vi "New.vi"(7 "CreateMethod(Create or look up existing)":T1(ring), 8 "error in (no error)":errorcluster, 10 "Object name":string, 11 "Websocket In":refnum<class "Websocket.lvclass">) -> (0 "error out":errorcluster, 1 "NewObjectCreated":bool, 2 "DVRRefOut":refnum<data-value>, 3 "Websocket Out":refnum<class "Websocket.lvclass">, 5 "ObjectQueueName":string)   [LabVIEW 2017, in "Front Panel Publisher.lvlib" / "Websocket.lvclass"]
uses:
  Websocket.lvclass
  Protected/Object Attributes.ctl
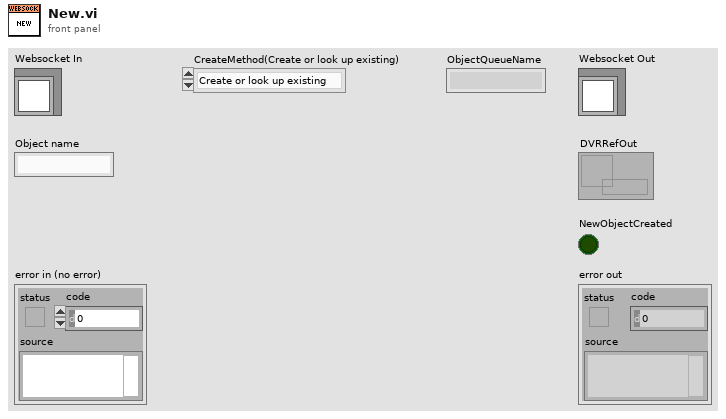
[diagram p1: front panel]
types:
  T1 = enum16{"Create or look up existing", "Look up existing"}
  T2 = typedef "Front Panel Publisher.lvlib/Websocket.lvclass/Object Attributes.ctl" = cluster{"Port":u16, "TCP Refs":refnum<k5>[], "Connection IDs":u64[]}
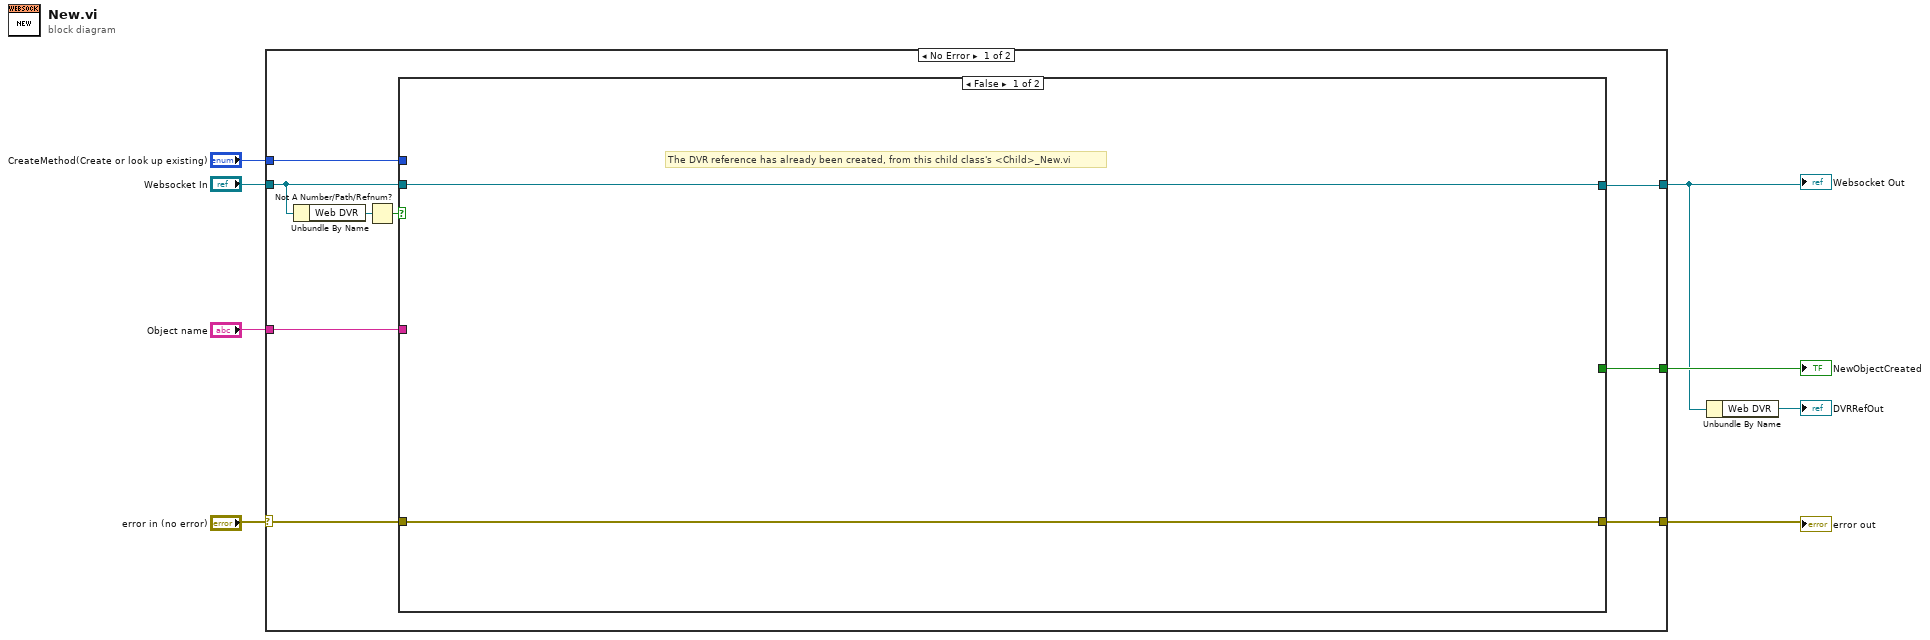
[diagram p0: block diagram]
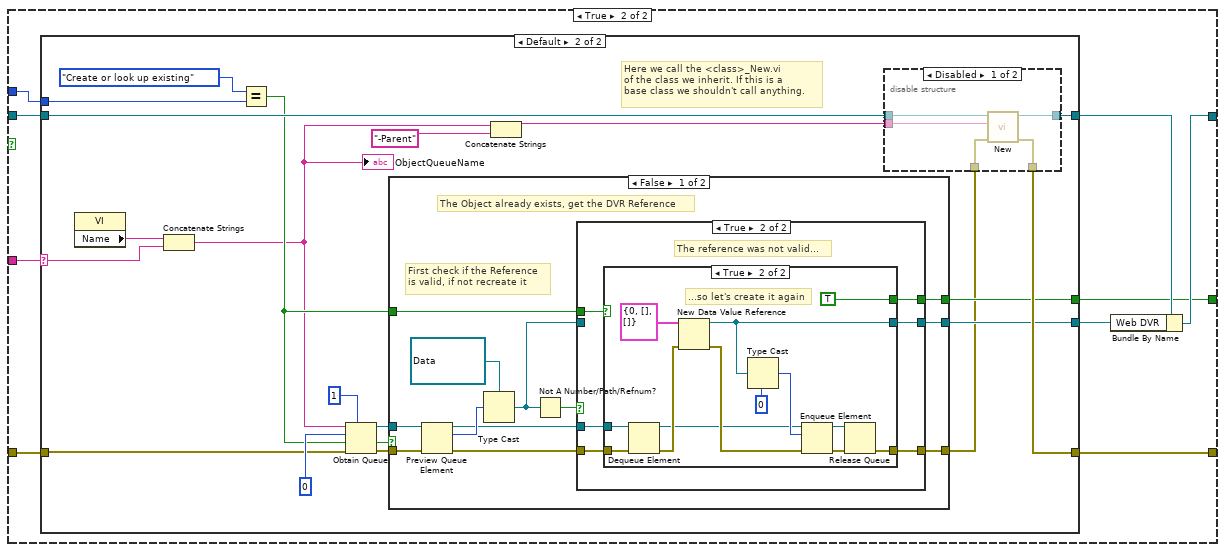
[diagram p2: hidden frame]
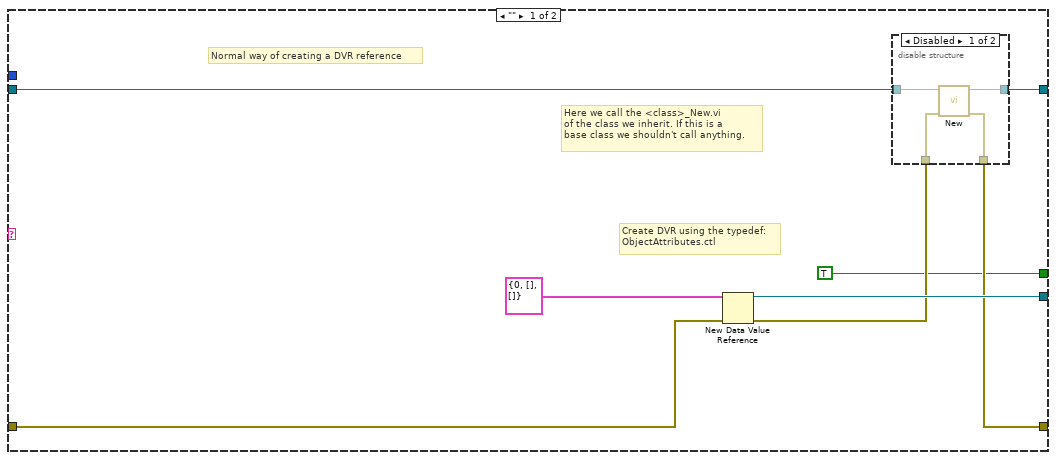
[diagram p3: hidden frame]
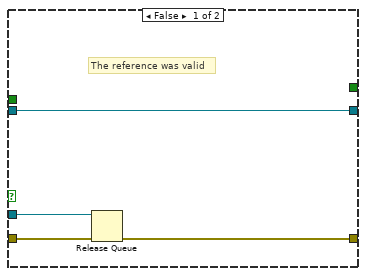
[diagram p5: hidden frame]
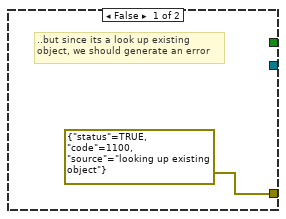
[diagram p6: hidden frame]
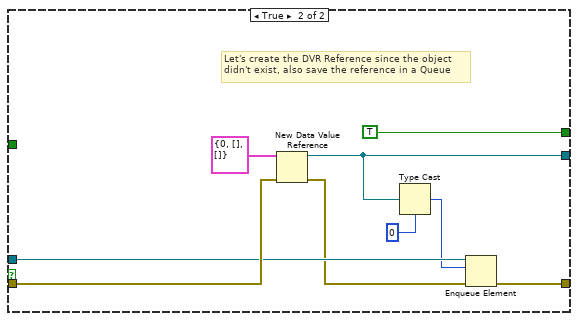
[diagram p7: hidden frame]
diagram:
  n1 = case shown="No Error" "error in (no error)" {
    selector: "error in (no error)" -> [w17 w116]
    tunnel: [w14 w116] -> w4
    tunnel: "CreateMethod(Create or look up existing)" -> [w15 _]
    tunnel: "Object name" -> [w16 _]
    tunnel: "Websocket In" -> [w13 w115]
    tunnel: [w12 w115] -> w2
    tunnel: [w11 _] -> w3
    frame No Error {
      n2 = Unbundle By Name(w13) -> ("Web DVR"=w10:refnum<data-value>)
      n3 = Not A Number/Path/Refnum?(number/path/refnum=w10) -> (NaN/Path/Refnum?=w9:bool)
      n4 = case shown="False" w9 {
        tunnel: w17 -> [w19 w28]
        tunnel: w16 -> [_ w27]
        tunnel: w15 -> [_ w26]
        tunnel: [w19 w25] -> w14
        tunnel: w13 -> [w18 w23]
        tunnel: [w18 w24] -> w12
        tunnel: [_ w21] -> w11
        frame False {
          # "The DVR reference has already been created, from this child class's <Child>_New.vi"
        }
        frame True {
          n5 = case shown="Default" w27 {
            selector: w27 -> [_ w54]
            tunnel: w28 -> [w36 w52]
            tunnel: [w31 w53] -> w25
            tunnel: w26 -> [_ w61]
            tunnel: [w35 w47] -> w20
            tunnel: w23 -> [w34 w60]
            tunnel: [w33 w59] -> w22
            tunnel: [TRUE w46] -> w21
            frame "" {
              # "Create DVR using the typedef:\nObjectAttributes.ctl"
              # "Here we call the <class>_New.vi\nof the class we inherit. If this is a\nbase class we shouldn't call anything."
              # "Normal way of creating a DVR reference"
              n6 = New Data Value Reference(data value=T2 {"Port"=0, "TCP Refs"=[], "Connection IDs"=[]} ("Data 2"), error in=w36) -> (data value reference=w35:refnum<data-value>, error out=w32:errorcluster)
              n7 = disable-structure shown="Disabled" {
                disable-tunnel: w34 -> [w40 w42]
                disable-tunnel: [w39 w42] -> w33
                disable-tunnel: w32 -> [w38 w41]
                disable-tunnel: [w37 w41] -> w31
                frame Disabled {
                  n8 = call "New.vi"("error in (no error)"=w38, "Websocket In"=w40) -> ("error out"=w37:errorcluster, "Websocket Out"=w39:refnum<class "Websocket.lvclass">)  [unwired: 5 in, 3 out]
                }
                frame Enabled {
                }
              }
            }
            frame Default {
              # "Here we call the <class>_New.vi\nof the class we inherit. If this is a\nbase class we shouldn't call anything."
              n9 = property class="VI"() -> ("Name"=w55:string)  [unwired: 2 in, 2 out]
              n10 = Concatenate Strings(w55, w54) -> (w43:string)
              "ObjectQueueName" <- w43
              n11 = Equal?(x=T1."Create or look up existing", y=w61) -> (x = y?=w48:bool)
              n12 = Obtain Queue(max queue size (-1, unlimited)=1, name (unnamed)=w43, element data type=u32 0 ("DataRef"), create if not found? (T)=w48, error in (no error)=w52) -> (queue out=w49:refnum<queue>, created new?=w50:bool, error out=w51:errorcluster)
              n13 = case shown="False" w50 {
                tunnel: w51 -> [w73 w107]
                tunnel: w49 -> [w74 w106]
                tunnel: [w69 w103] -> w45
                tunnel: [w67 w102] -> w47
                tunnel: [w65 TRUE] -> w46
                tunnel: w48 -> [w64 _]
                frame False {
                  # "First check if the Reference\nis valid, if not recreate it"
                  # "The Object already exists, get the DVR Reference"
                  n14 = Preview Queue Element(queue=w74, error in (no error)=w73) -> (queue out=w66:refnum<queue>, element=w72:u32, error out=w71:errorcluster)  [unwired: 1 in, 1 out]
                  n15 = Type Cast(type=refnum<data-value> refnum ("DVRRef(Hidden)"), x=w72) -> (*(type *) &x=w68:refnum<data-value>)
                  n16 = Not A Number/Path/Refnum?(number/path/refnum=w68) -> (NaN/Path/Refnum?=w70:bool)
                  n17 = case shown="True" w70 {
                    tunnel: w71 -> [w75 w83]
                    tunnel: [w76 w81] -> w69
                    tunnel: w68 -> [w78 _]
                    tunnel: [w78 w82] -> w67
                    tunnel: w66 -> [w77 w84]
                    tunnel: [_ w80] -> w65
                    tunnel: w64 -> [_ w79]
                    frame False {
                      # "The reference was valid"
                      n18 = Release Queue(queue=w77, error in (no error)=w75) -> (error out=w76:errorcluster)  [unwired: 1 in, 2 out]
                    }
                    frame True {
                      # "The reference was not valid..."
                      n19 = case shown="True" w79 {
                        tunnel: w84 -> [_ w98]
                        tunnel: w83 -> [_ w97]
                        tunnel: [_ w91] -> w82
                        tunnel: [errorcluster {"status"=TRUE, "code"=1100, "source"="looking up existing object"} ("error out") w87] -> w81
                        tunnel: [_ TRUE] -> w80
                        frame False {
                          # "..but since its a look up existing\nobject, we should generate an error"
                        }
                        frame True {
                          # "...so let's create it again"
                          n20 = Dequeue Element(queue=w98, error in (no error)=w97) -> (queue out=w92:refnum<queue>, error out=w94:errorcluster)  [unwired: 1 in, 2 out]
                          n21 = New Data Value Reference(data value=T2 {"Port"=0, "TCP Refs"=[], "Connection IDs"=[]} ("Data"), error in=w94) -> (data value reference=w91:refnum<data-value>, error out=w93:errorcluster)
                          n22 = Type Cast(type=u32 0 ("ObjectQueue"), x=w91) -> (*(type *) &x=w95:u32)
                          n23 = Enqueue Element(queue=w92, element=w95, error in (no error)=w93) -> (queue out=w88:refnum<queue>, error out=w89:errorcluster)  [unwired: 1 in, 1 out]
                          n24 = Release Queue(queue=w88, error in (no error)=w89) -> (error out=w87:errorcluster)  [unwired: 1 in, 2 out]
                        }
                      }
                    }
                  }
                }
                frame True {
                  # "Let's create the DVR Reference since the object\ndidn't exist, also save the reference in a Queue"
                  n25 = New Data Value Reference(data value=T2 {"Port"=0, "TCP Refs"=[], "Connection IDs"=[]} ("Data"), error in=w107) -> (data value reference=w102:refnum<data-value>, error out=w104:errorcluster)
                  n26 = Type Cast(type=u32 0 ("ObjectQueue"), x=w102) -> (*(type *) &x=w101:u32)
                  n27 = Enqueue Element(queue=w106, element=w101, error in (no error)=w104) -> (error out=w103:errorcluster)  [unwired: 1 in, 2 out]
                }
              }
              n28 = Concatenate Strings(w43, "-Parent" ("string")) -> (w56:string)
              n29 = disable-structure shown="Disabled" {
                disable-tunnel: w60 -> [w112 w114]
                disable-tunnel: [w111 w114] -> w59
                disable-tunnel: w56 -> [w110 _]
                disable-tunnel: w45 -> [w109 w113]
                disable-tunnel: [w108 w113] -> w53
                frame Disabled {
                  n30 = call "New.vi"("error in (no error)"=w109, "Object name"=w110, "Websocket In"=w112) -> ("error out"=w108:errorcluster, "Websocket Out"=w111:refnum<class "Websocket.lvclass">)  [unwired: 4 in, 3 out]
                }
                frame Enabled {
                }
              }
            }
          }
          n31 = Bundle By Name(cluster=w22, "Web DVR"=w20) -> (w24:refnum<class "Websocket.lvclass">)
        }
      }
    }
    frame Error {
    }
  }
  "error out" <- w4
  "Websocket Out" <- w2
  "NewObjectCreated" <- w3
  n32 = Unbundle By Name(w2) -> ("Web DVR"=→"DVRRefOut":refnum<data-value>)
